vi "7-OCU Jaime.vi"() -> ()   [LabVIEW 2010]
uses:
  6-OCU Neurons/MainControls.ctl
  6-OCU Neurons/MainIndicators.ctl
  4-High Neurons/4.4-How Sensor Typedef.ctl
  6-OCU Neurons/6.1-UDP Saitek.ctl
  7-OCU/TabEnum.ctl
  7-OCU/7.0-Global.vi
panel:
  out "ManualMode":bool
  out "7.7.2 Main Indicators":T1
  in  "Stop Loops":bool
  out "Startup&Shutdown":bool
  out "Main Tab":string
  in  "Main Tab Interface":T3
  in  "IP address of Forebrain":string="127.0.0.1"
  out "Process loop":bool
  out "Drive Motor Check":bool
  out "Steer Motor Check":bool
  out "LIDAR Motor Check":bool
  out "Vector Nav Check":bool
  in  "Saitek Controler":T4 {"Right" scale=-32767.0..32767.0; "Left" scale=-32767.0..32767.0; "Yaw" scale=-32767.0..32767.0; "Roll" scale=-32767.0..32767.0; "Pitch" scale=-32767.0..32767.0}
  out "Stop Saitek":bool
  out "Dashboard":T5 {"Battery" scale=0.0..24.0; "Heading" scale=-180.0..180.0; "Speed" scale=0.0..10.0}
  in  "7.7.1 AutoModeDatums":T6
  out "7.7.2 Main Indicators 2":T1
  in  "Start/Stop Mission":bool
  out "Hearbeat":bool
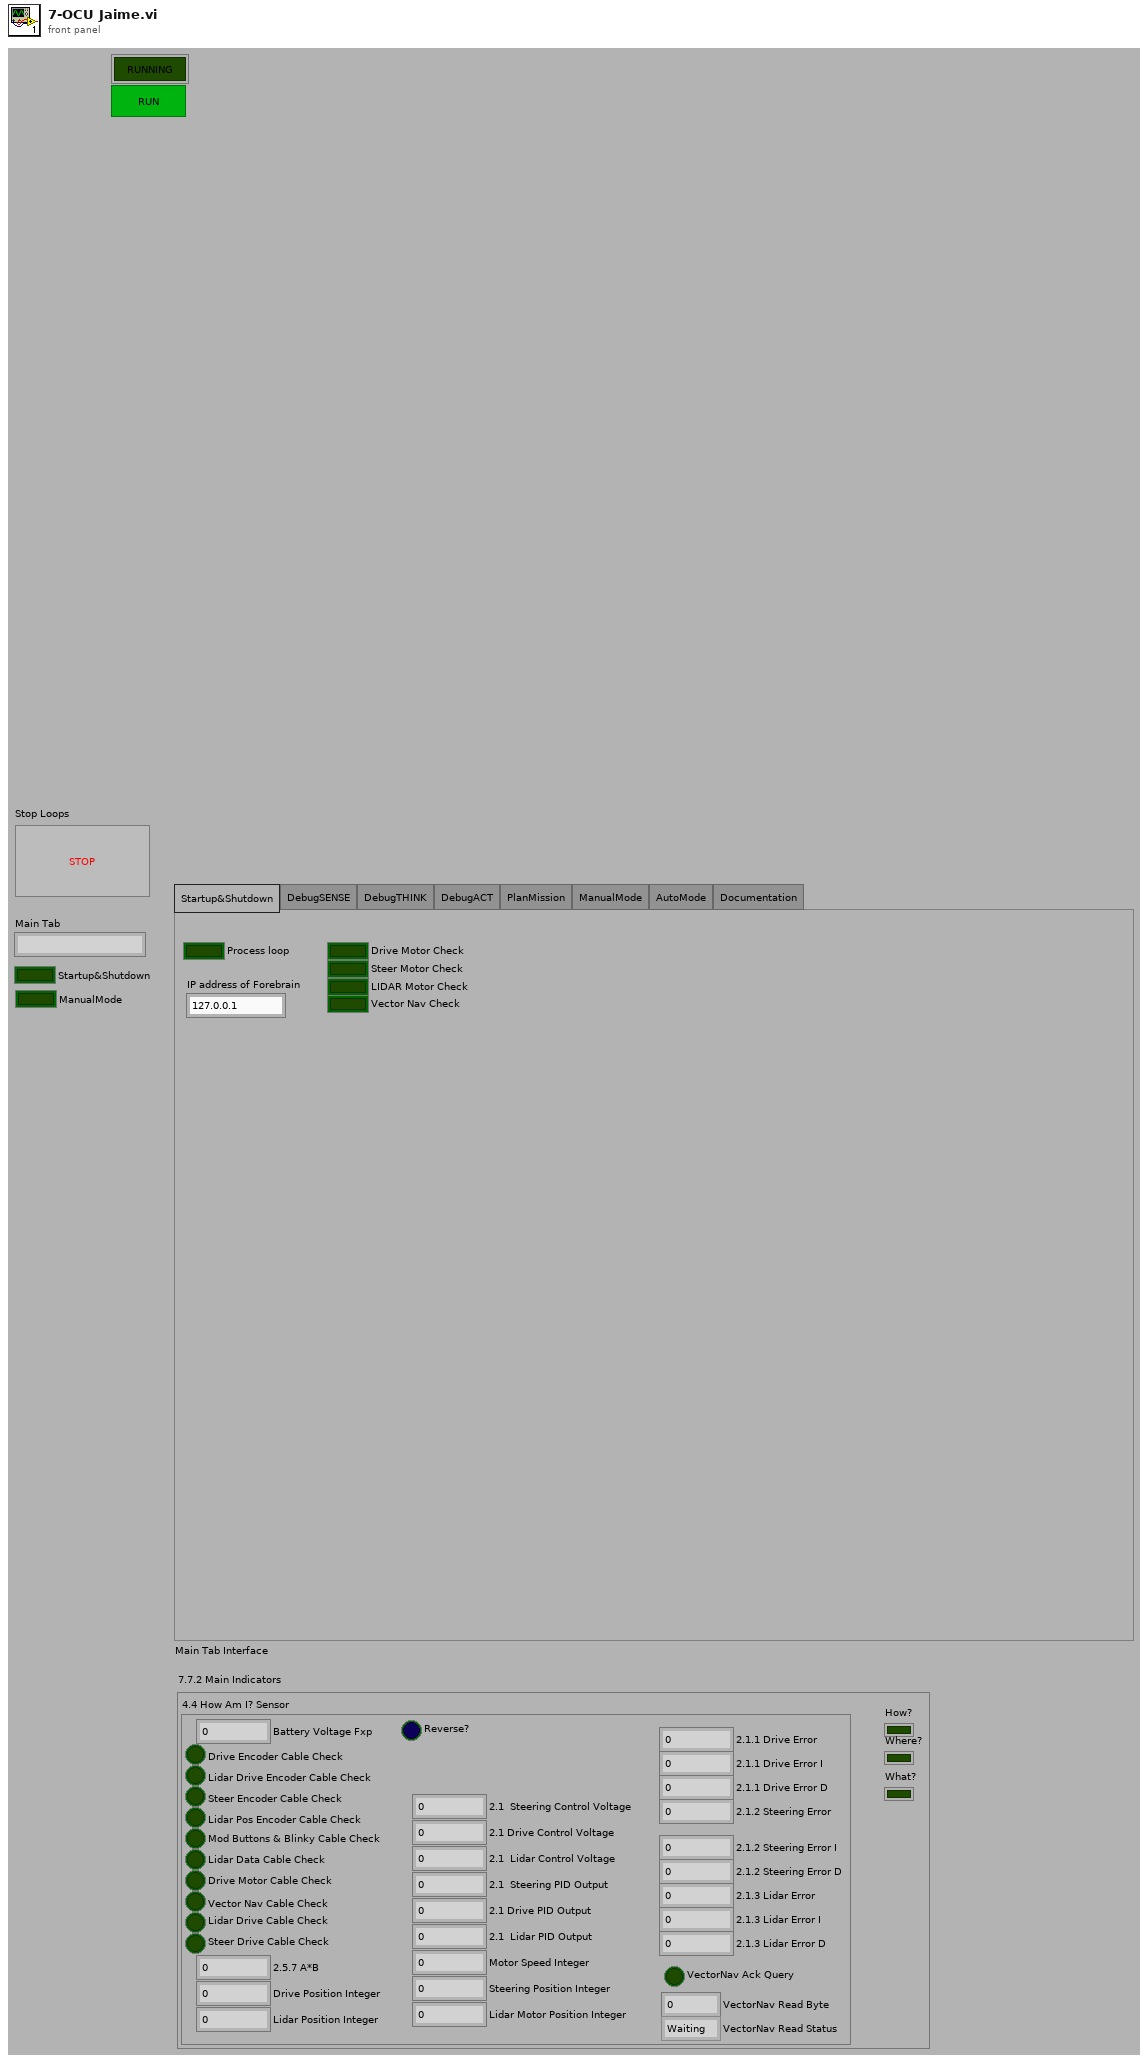
[diagram p1: front panel]
types:
  T1 = typedef "MainIndicators.ctl" = cluster{"4.4 How Am I? Sensor":T2, "How?":bool, "Where?":bool, "What?":bool}
  T2 = typedef "4.4-How Sensor Typedef.ctl" = cluster{"Motor Speed Integer":i32, "Drive Position Integer":i32, "Lidar Position Integer":i32, "Lidar Motor Position Integer":i32, "Steering Position Integer":i32, "Battery Voltage Fxp":dbl, "Drive Encoder Cable Check":bool, "Lidar Drive Encoder Cable Check":bool, "Steer Encoder Cable Check":bool, "Lidar Pos Encoder Cable Check":bool, "Mod Buttons & Blinky Cable Check":bool, "Lidar Data Cable Check":bool, "Drive Motor Cable Check":bool, "Vector Nav Cable Check":bool, "Lidar Drive Cable Check":bool, "Steer Drive Cable Check":bool, "Reverse?":bool, "2.1  Steering Control Voltage":dbl, "2.1 Drive Control Voltage":dbl, "2.1  Lidar Control Voltage":dbl, "2.5.7 A*B":dbl, "2.1  Steering PID Output":dbl, "2.1 Drive PID Output":dbl, "2.1  Lidar PID Output":dbl, "2.1.1 Drive Error":dbl, "2.1.1 Drive Error I":dbl, "2.1.1 Drive Error D":dbl, "2.1.2 Steering Error":dbl, "2.1.2 Steering Error I":dbl, "2.1.2 Steering Error D":dbl, "2.1.3 Lidar Error":dbl, "2.1.3 Lidar Error I":dbl, "2.1.3 Lidar Error D":dbl, "VectorNav Ack Query":bool, "VectorNav Read Byte":u8, "VectorNav Read Status":enum16{"Waiting", "Reading", "Done"}}
  T3 = typedef "TabEnum.ctl" = enum32{"Startup&Shutdown", "DebugSENSE", "DebugTHINK", "DebugACT", "PlanMission", "ManualMode", "AutoMode", "Documentation"}
  T4 = typedef "6.1-UDP Saitek.ctl" = cluster{"Trig":bool, "2":bool, "3":bool, "4":bool, "5":bool, "6":bool, "7":bool, "8":bool, "9":bool, "10":bool, "11":bool, "Pitch":i32, "Ang":bool[], "Wheel":dbl, "Roll":i32, "Yaw":i32, "Left":i32, "Right":i32}
  T5 = cluster{"Speed":dbl, "Heading":dbl, "Battery":dbl, "Time":dbl}
  T6 = typedef "MainControls.ctl" = cluster{"RunAutoMode":bool, "Rerun MDF":bool, "Pause":bool}
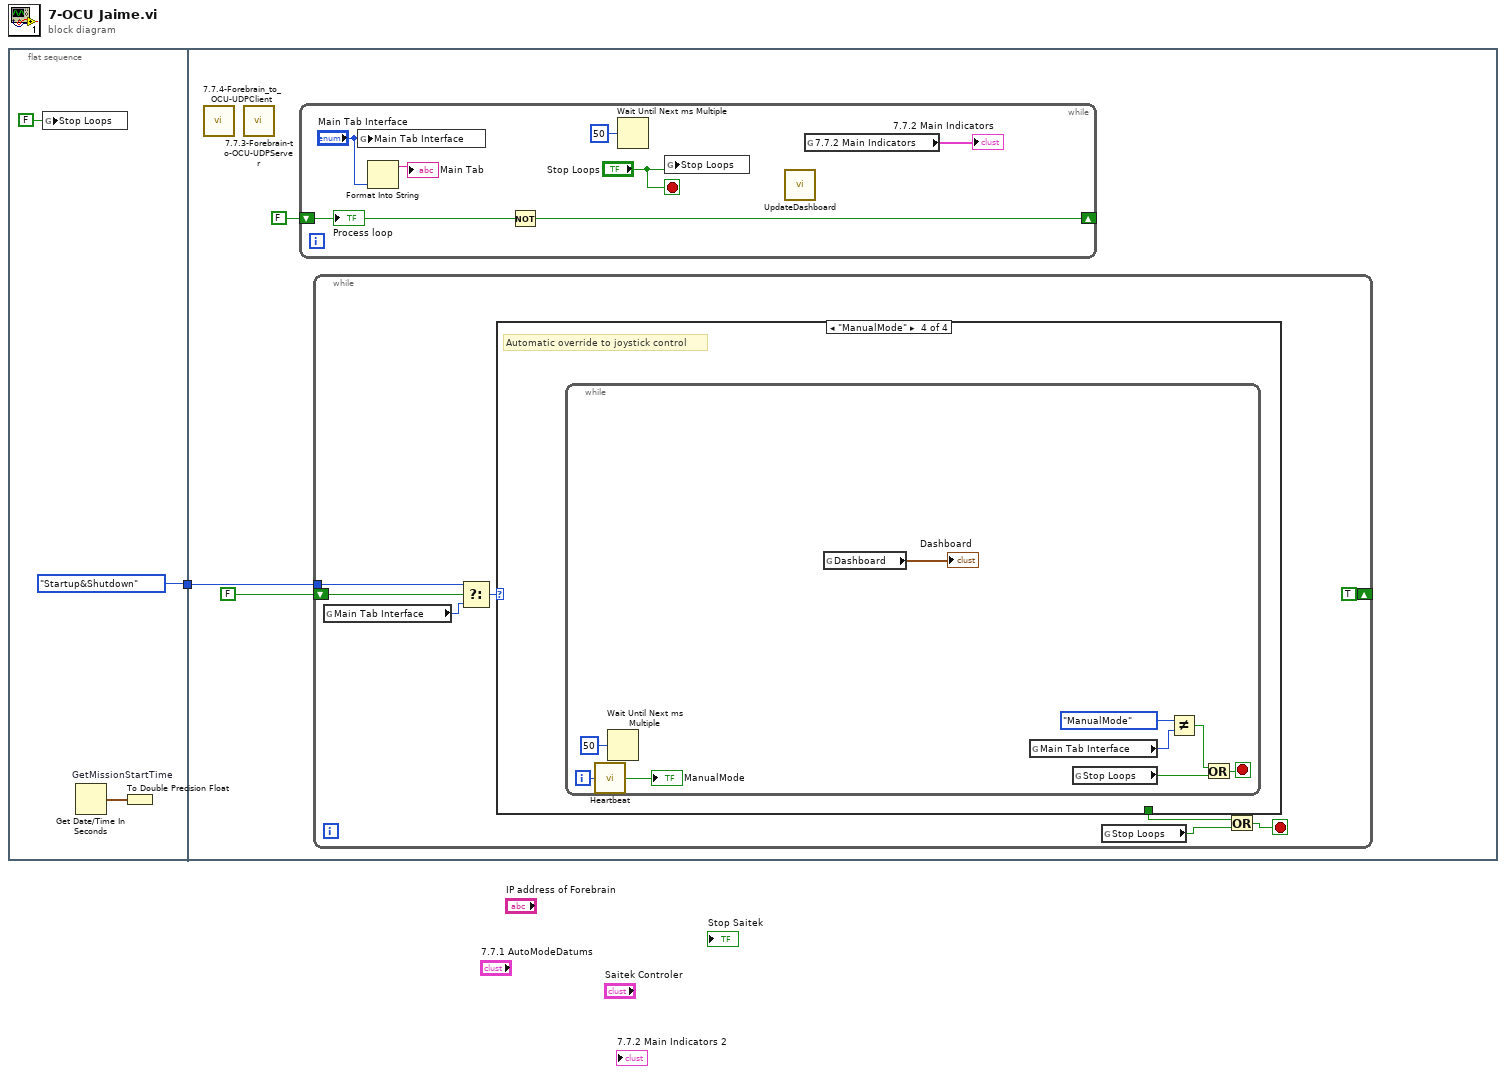
[diagram p0: block diagram]
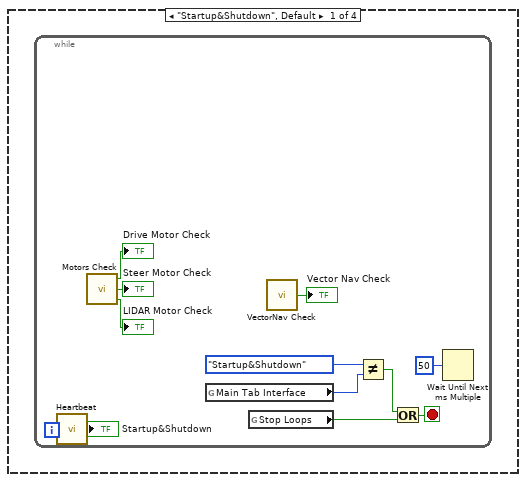
[diagram p2: hidden frame]
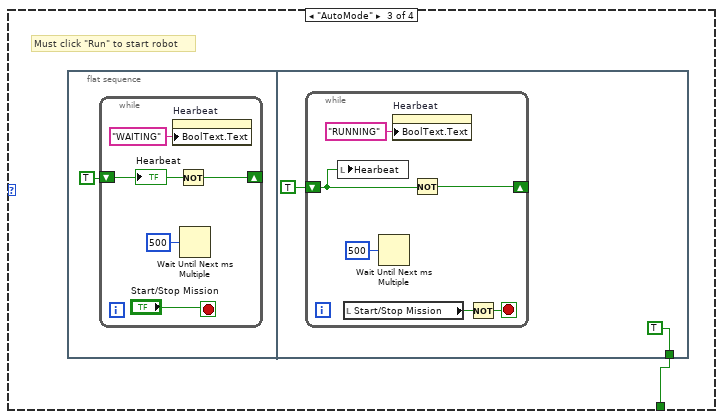
[diagram p4: hidden frame]
diagram:
  n1 = flat-sequence {
    tunnel: [TabEnum."Startup&Shutdown" ("Main Tab Interface  2")] -> w1
    tunnel: w1 -> [w7]
    frame #0 {
      n2 = global write "7.0-Global.vi" "Stop Loops"(FALSE ("Stop Loops")) -> ()
      n3 = Get Date/Time In Seconds "GetMissionStartTime"() -> (seconds since 1Jan1904=w4:timestamp)
      n4 = To Double Precision Float(number=w4) -> ()  [unwired: 1 out]
    }
    frame #1 {
      n5 = call "7.7.4-Forebrain_to_OCU-UDPClient.vi"() -> ()  [unwired: 1 in]
      n6 = call "7.7.3-Forebrain-to-OCU-UDPServer.vi"() -> ()  [unwired: 1 in]
      n7 = while {
        shift-right: [w13] -> _
        shift-left: FALSE -> [w14]
        stop <- "Stop Loops" stop-if-true
        n8 = global write "7.0-Global.vi" "Main Tab Interface"("Main Tab Interface") -> ()
        n9 = Format Into String("Main Tab Interface") -> (resulting string=→"Main Tab":string)  [unwired: 3 in, 1 out]
        n10 = Not(x=w14) -> (.not. x?=w13:bool)
        n11 = Wait Until Next ms Multiple(millisecond multiple=u32 50) -> ()  [unwired: 1 out]
        n12 = global write "7.0-Global.vi" "Stop Loops"("Stop Loops") -> ()
        n13 = call "UpdateDashboard.vi"() -> ()  [unwired: 12 in]
        n14 = global read "7.0-Global.vi" "7.7.2 Main Indicators"() -> (→"7.7.2 Main Indicators":T1)
        "Process loop" <- w14
      }
      n15 = while {
        shift-right: [TRUE] -> _
        shift-left: FALSE -> [w18]
        tunnel: w7 -> [w20]
        stop <- w21 stop-if-true
        n16 = global read "7.0-Global.vi" "Main Tab Interface"() -> (w16:T3)
        n17 = Select(t=w20, s=w18, f=w16) -> (s? t:f=w19:T3)
        n18 = case shown="\"ManualMode\"" w19 {
          tunnel: [_ _ w35 _] -> w22
          frame "Startup&Shutdown", Default {
            n19 = while {
              i -> [w24]
              stop <- w33 stop-if-true
              n20 = call "Heartbeat.vi"("Loop Iteration"=w24) -> ("Running?"=→"Startup&Shutdown":bool)
              n21 = call "Motors Check.vi"() -> ("LIDAR Motor Check"=→"LIDAR Motor Check":bool, "Steer Motor Check"=→"Steer Motor Check":bool, "Drive Motor Check"=→"Drive Motor Check":bool)  [unwired: 4 in]
              n22 = global read "7.0-Global.vi" "Main Tab Interface"() -> (w31:T3)
              n23 = global read "7.0-Global.vi" "Stop Loops"() -> (w34:bool)
              n24 = call "VectorNav Check.vi"() -> ("Vector Nav Check"=→"Vector Nav Check":bool)  [unwired: 1 in]
              n25 = Not Equal?(x=TabEnum."Startup&Shutdown" ("Main Tab Interface  2"), y=w31) -> (x != y?=w32:bool)
              n26 = Or(x=w32, y=w34) -> (x .or. y?=w33:bool)
              n27 = Wait Until Next ms Multiple(millisecond multiple=u32 50) -> ()  [unwired: 1 out]
            }
          }
          frame "PlanMission" {
            # "Either load MDF test or click on map"
          }
          frame "AutoMode" {
            # "Must click \"Run\" to start robot"
            n28 = flat-sequence {
              tunnel: [TRUE] -> w35
              frame #0 {
                n29 = while {
                  shift-right: [w39] -> _
                  shift-left: TRUE -> [w40]
                  stop <- "Start/Stop Mission" stop-if-true
                  n30 = property on="Hearbeat" class="Bool"("BoolText.Text"="WAITING" ("Boolean Text.Text")) -> ()  [unwired: 2 in, 2 out]
                  n31 = Not(x=w40) -> (.not. x?=w39:bool)
                  n32 = Wait Until Next ms Multiple(millisecond multiple=u32 500) -> ()  [unwired: 1 out]
                  "Hearbeat" <- w40
                }
              }
              frame #1 {
                n33 = while {
                  shift-right: [w49] -> _
                  shift-left: TRUE -> [w44]
                  stop <- w46 stop-if-true
                  n34 = local write "Hearbeat"(w44) -> ()
                  n35 = local read "Start/Stop Mission"() -> (w47:bool)
                  n36 = Wait Until Next ms Multiple(millisecond multiple=u32 500) -> ()  [unwired: 1 out]
                  n37 = property on="Hearbeat" class="Bool"("BoolText.Text"="RUNNING" ("Boolean Text.Text")) -> ()  [unwired: 2 in, 2 out]
                  n38 = Not(x=w44) -> (.not. x?=w49:bool)
                  n39 = Not(x=w47) -> (.not. x?=w46:bool)
                }
              }
            }
          }
          frame "ManualMode" {
            # "Automatic override to joystick control"
            n40 = while {
              i -> [w51]
              stop <- w57 stop-if-true
              n41 = call "Heartbeat.vi"("Loop Iteration"=w51) -> ("Running?"=→"ManualMode":bool)
              n42 = Wait Until Next ms Multiple(millisecond multiple=u32 50) -> ()  [unwired: 1 out]
              n43 = global read "7.0-Global.vi" "Dashboard"() -> (→"Dashboard":T5)
              n44 = global read "7.0-Global.vi" "Main Tab Interface"() -> (w55:T3)
              n45 = global read "7.0-Global.vi" "Stop Loops"() -> (w58:bool)
              n46 = Not Equal?(x=TabEnum."ManualMode" ("Main Tab Interface  2"), y=w55) -> (x != y?=w56:bool)
              n47 = Or(x=w56, y=w58) -> (x .or. y?=w57:bool)
            }
          }
        }
        n48 = global read "7.0-Global.vi" "Stop Loops"() -> (w15:bool)
        n49 = Or(x=w22, y=w15) -> (x .or. y?=w21:bool)
      }
    }
  }
